vi "H5Fclose.vi"(8 "error in (no error)":errorcluster, 11 "file_id":i32) -> (0 "error out":errorcluster, 3 "status":i32)   [LabVIEW 2009]
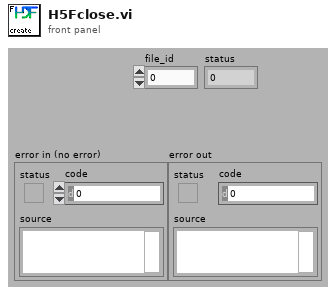
[diagram p1: front panel]
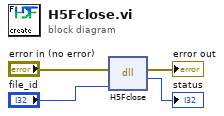
[diagram p0: block diagram]
diagram:
  n1 = dll-call lib="hdf5dll" fn="H5Fclose"(error in="error in (no error)", "file_id"="file_id") -> (error out=→"error out":errorcluster, "return type"=→"status":i32)  [unwired: 3 in, 1 out]
